vi "Motor3_ESC.vi"(8 "error in (no error)":errorcluster, 10 "Percent Power":dbl format="%#_13g", 11 "Channel Name":tag="B/PWM1") -> (0 "error out":errorcluster)   [LabVIEW 2019]
doc: "The myRIO Project template acquires acceleration data from the onboard accelerometer and displays the changes of acceleration values in a waveform chart."
uses:
  <vilib>/Utility/error.llb/Error Cluster From Error Code.vi
  <vilib>/myRIO/Common/Instrument Driver Framework/myRIO v1.0/PWM/vis/myRIO v1.0 Write PWM.vi
  <vilib>/myRIO/Instrument Drivers/Onboard IO/PWM/PWM.lvlib
panel:
  # "For a frequency of 120 Hz, the esc will respond to a duty cycle of btwn ~0.1 and ~0.25. Double the frequency to double the response range (240 Hz will respond to ~.2 to ~.5)."
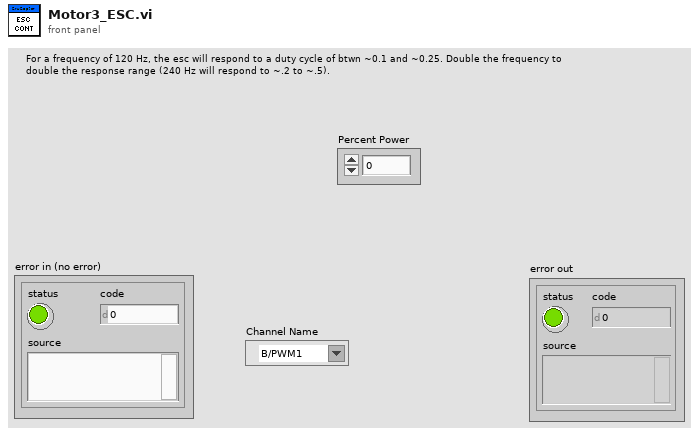
[diagram p1: front panel]
types:
  T1 = typedef "PWM.lvlib/PWM Reference.ctl" = cluster{"myRIO Reference":T2, "PWM Channels Enum":T6, "PWM Configuration":T7}
  T2 = typedef "myRIO Generic Hardware Reference.ctl" = cluster{"myRIO Model":T3, "myRIO Hardware Reference":T4}
  T3 = typedef "Hardware Version Enum.ctl" = enum16{"Unknown", "myRIO-1900", "myRIO-1950", "roboRIO", "NI ELVIS RIO CM", "ELVIS III"}
  T4 = typedef "myRIO v1.0 Reference.ctl" = cluster{"Generic FPGA Reference":T5, "Allow multiple opens":bool}
  T5 = typedef "Generic FPGA Reference.ctl" = refnum<k20>
  T6 = typedef "PWM Channels Enum.ctl" = enum16{"Not Connected", "C/PWM0", "C/PWM1", "A/PWM0", "A/PWM1", "A/PWM2", "A/PWM3", "A/PWM4", "A/PWM5", "A/PWM6", "A/PWM7", "A/PWM8", "A/PWM9", "A/PWM10", "A/PWM11", "A/PWM12", "A/PWM13", "A/PWM14", "A/PWM15", "A/PWM16", "A/PWM17", "A/PWM18", "A/PWM19", "B/PWM0", "B/PWM1", "B/PWM2", "B/PWM3", "B/PWM4", "B/PWM5", "B/PWM6", "B/PWM7", "B/PWM8", "B/PWM9", "B/PWM10", "B/PWM11", "B/PWM12", "B/PWM13", "B/PWM14", "B/PWM15", "B/PWM16", "B/PWM17", "B/PWM18", "B/PWM19", "PWM/PWM0", "PWM/PWM1", "PWM/PWM2", "PWM/PWM3", "PWM/PWM4", "PWM/PWM5", "PWM/PWM6", "PWM/PWM7", "PWM/PWM8", "PWM/PWM9"}
  T7 = typedef "PWM.lvlib/PWM Configuration.ctl" = cluster{"Frequency":dbl, "Duty Cycle":dbl}
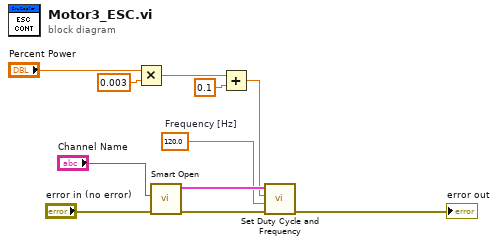
[diagram p0: block diagram]
diagram:
  w8 = 120.0  # Frequency [Hz]
  n1 = Multiply(x="Percent Power", y=0.003) -> (x*y=w4:dbl)
  n2 = call <vilib>:"Smart Open.vi"("error in (no error)"="error in (no error)", "Channel Name"="Channel Name") -> ("error out"=w9:errorcluster, "PWM Ref Out"=w10:T1)  [unwired: 8 in]
  n3 = Add(x=w4, y=0.1) -> (x+y=w2:dbl)
  n4 = call <vilib>:"Set Duty Cycle and Frequency.vi"("error in (no error)"=w9, "Frequency [Hz]"=w8, "Duty Cycle"=w2, "PWM Ref In"=w10) -> ("error out"=→"error out":errorcluster)  [unwired: 5 in, 1 out]
